vi "Phasor Get Valid Time Gate Location.vi"(8 "Period":dbl, 9 "X":dbl, 10 "Min X":dbl, 11 "Max X":dbl) -> (1 "X in [Min X, Max X]":dbl)   [LabVIEW 2021, in "Phasor.lvlib"]
uses:
  Phasor.lvlib
  c3d34567-bea7-48b7-ba1e-b930059b104d.vi
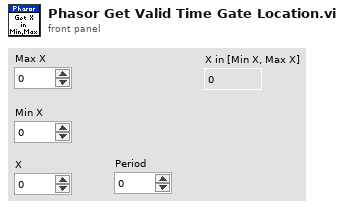
[diagram p1: front panel]
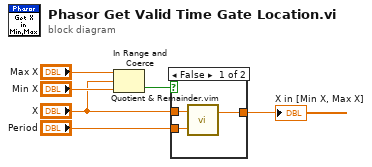
[diagram p0: block diagram]
diagram:
  n1 = In Range and Coerce(upper limit="Max X", x="X", lower limit="Min X") -> (In Range?=w1:bool)  [unwired: 1 out]
  n2 = case shown="False" w1 {
    tunnel: "X" -> [w9 w10]
    tunnel: "Period" -> [w7 _]
    tunnel: [w8 w10] -> w2
    frame False {
      n3 = call "Quotient & Remainder.vim"("y"=w7, "x"=w9) -> ("x - E(x/y)y"=w8:dbl)  [unwired: 1 out]
    }
    frame True {
    }
  }
  "X in [Min X, Max X]" <- w2
